vi "Inverse f Filter (CDB).vi"(6 "unity gain freq (rad/s)":dbl=1.0 format="%.2g", 7 "reset":bool, 8 "filter specifications":T3={"lower cutoff freq"=0.1, "higher cutoff freq"=100.0, "order"=5}, 9 "exponent":dbl=1.0 format="%.2g", 10 "fs":dbl=1000.0 format="%.2f", 11 "X":cdb[](array[numeric])) -> (0 "error":i32, 1 "magnitude error (dB)":T1, 2 "filter information":T2, 3 "Filtered X":cdb[](array[numeric]), 4 "noise bandwidth":dbl=1.0 format="%.2g")   [LabVIEW 2020, in "NI_AALBase.lvlib"]
doc: "Designs and implements an IIR filter whose magnitude-squared response is inversely proportional to frequency over a specified frequency range. This inverse-f filter is typically used to colorize spectrally flat, or white, noise. Wire data to the <B>X</B> input to determine the polymorphic instance to use or manually select the instance."
uses:
  NI_AALBase.lvlib
  IIR Cascade Filter (CDB).vi
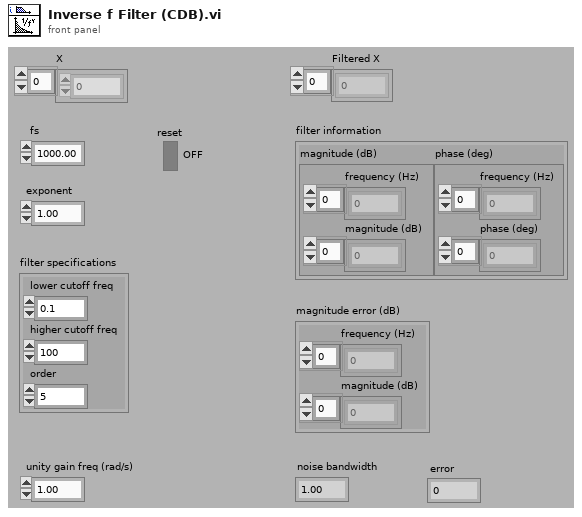
[diagram p1: front panel]
types:
  T1 = cluster{"frequency (Hz)":dbl[], "magnitude (dB)":dbl[]}
  T2 = cluster{"magnitude (dB)":cluster{"frequency (Hz)":dbl[], "magnitude (dB)":dbl[]}, "phase (deg)":cluster{"frequency (Hz)":dbl[], "phase (deg)":dbl[]}}
  T3 = cluster{"lower cutoff freq":dbl, "higher cutoff freq":dbl, "order":i32}
  T4 = cluster{"filter structure":enum32{"IIR 2nd Order", "IIR 4th Order"}, "Reverse Coefficients":dbl[], "Forward Coefficients":dbl[]}
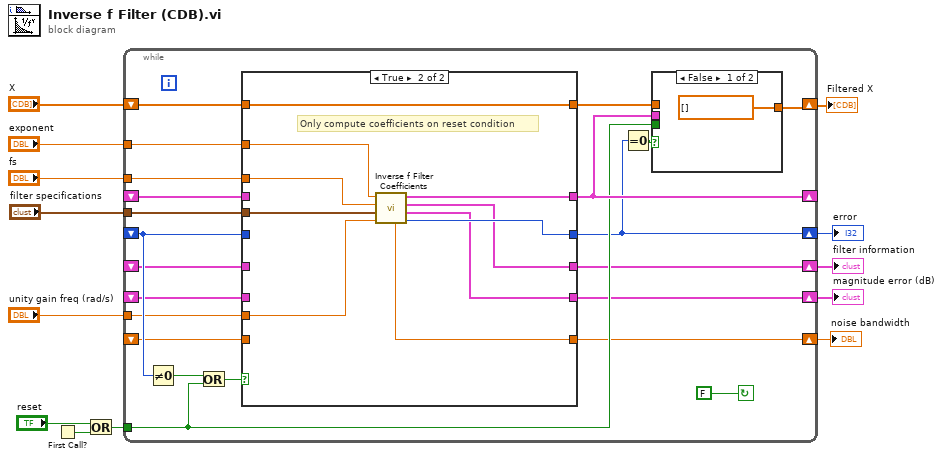
[diagram p0: block diagram]
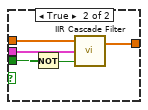
[diagram p2: hidden frame]
diagram:
  n1 = First Call?() -> (First Call?: T/F=w8:bool)
  n2 = Or(x="reset", y=w8) -> (x .or. y?=w7:bool)
  n3 = while {
    tunnel: w7 -> [w25]
    shift-left: _ -> [w33]
    shift-right: [w34] -> _
    tunnel: "exponent" -> [w30]
    tunnel: "fs" -> [w29]
    tunnel: "filter specifications" -> [w28]
    shift-right: [w23] -> w10
    shift-left: _ -> [w26]
    shift-right: [w21] -> w2
    shift-left: _ -> [w20]
    shift-right: [w19] -> w1
    shift-left: _ -> [w18]
    tunnel: "unity gain freq (rad/s)" -> [w17]
    shift-right: [w16] -> w6
    shift-left: _ -> [w15]
    shift-right: [w14] -> w12
    shift-left: "X" -> [w32]
    stop <- FALSE continue-if-true
    n4 = Not Equal To 0?(x=w26) -> (x != 0?=w27:bool)
    n5 = Or(x=w27, y=w25) -> (x .or. y?=w24:bool)
    n6 = case shown="True" w24 {
      tunnel: [w47 w56] -> w34
      tunnel: w33 -> [w47 _]
      tunnel: w32 -> [w46 w57]
      tunnel: [w46 w57] -> w31
      tunnel: w30 -> [_ w55]
      tunnel: w29 -> [_ w48]
      tunnel: w28 -> [_ w49]
      tunnel: [w45 w54] -> w23
      tunnel: w26 -> [w45 _]
      tunnel: [w44 w53] -> w21
      tunnel: w20 -> [w44 _]
      tunnel: [w43 w52] -> w19
      tunnel: w18 -> [w43 _]
      tunnel: w17 -> [_ w50]
      tunnel: [w42 w51] -> w16
      tunnel: w15 -> [w42 _]
      frame False {
      }
      frame True {
        # "Only compute coefficients on reset condition"
        n7 = call "Inverse f Filter Coefficients.vi"("unity gain freq (rad/s)"=w50, "filter specifications"=w49, "fs"=w48, "exponent"=w55) -> ("error"=w54:i32, "magnitude error (dB)"=w52:T1, "filter information"=w53:T2, "IIR Filter Cluster"=w56:T4, "noise bandwidth"=w51:dbl)  [unwired: 3 in]
      }
    }
    n8 = Equal To 0?(x=w23) -> (x = 0?=w22:bool)
    n9 = case shown="False" w22 {
      tunnel: w34 -> [_ w41]
      tunnel: w31 -> [_ w40]
      tunnel: [cdb[] [] ("Filtered X") w39] -> w14
      tunnel: w25 -> [_ w37]
      frame False {
      }
      frame True {
        n10 = Not(x=w37) -> (.not. x?=w38:bool)
        n11 = call-poly "IIR Cascade Filter.vi"("init/cont (init:F)"=w38, "IIR Filter Cluster"=w41, "X"=w40) -> ("Filtered X"=w39:cdb[])  [unwired: 1 out]
      }
    }
  }
  "Filtered X" <- w12
  "error" <- w10
  "noise bandwidth" <- w6
  "filter information" <- w2
  "magnitude error (dB)" <- w1
